vi "Insert_test.vi"(7 "Added time":refnum<vi>, 8 "error in (no error)":errorcluster, 9 "Sorted hits":T2, 10 "Bottom hit charts":T1, 11 "Top hit charts":T1) -> (0 "error out":errorcluster)   [LabVIEW 2016]
uses:
  Typedefs/Hit chart cluster refnum.ctl
  Global Variables/Global Resolution.vi
panel:
  out "Numeric":u64
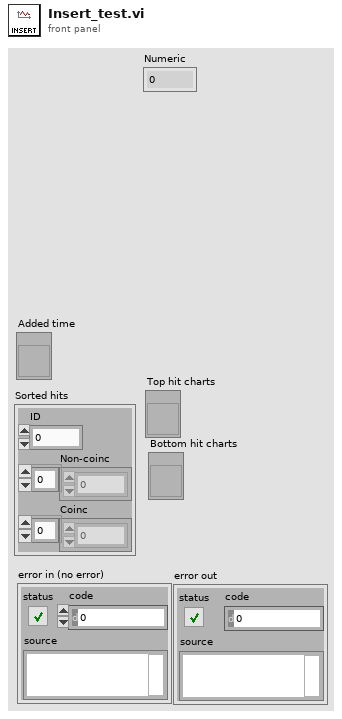
[diagram p1: front panel]
types:
  T1 = typedef "Hit chart cluster refnum.ctl" = refnum<vi>
  T2 = cluster{"ID":i8, "Non-coinc":u64[], "Coinc":u64[]}
  T3 = typedef "HitChart refnum.ctl" = refnum<vi>
  T4 = typedef "HitChart.ctl" = cluster{"Waveform Chart":cluster{"Coincidences":dbl, "Non-coincidences":dbl, "Ratio":dbl, "Total hits":dbl}[], "Last update timestamp":timestamp, "Resolution(s)":dbl, "nondisplayed coincs":i32, "nondisplayed noncoincs":i32, "Last upd":i64, "ID":i8}
  T5 = cluster{"Coincidences":dbl, "Non-coincidences":dbl, "Ratio":dbl, "Total hits":dbl}
  T6 = cluster{"Coincidences":dbl, "Non-coincidences":dbl, "Ratio":dbl, "Total hits":dbl}[]
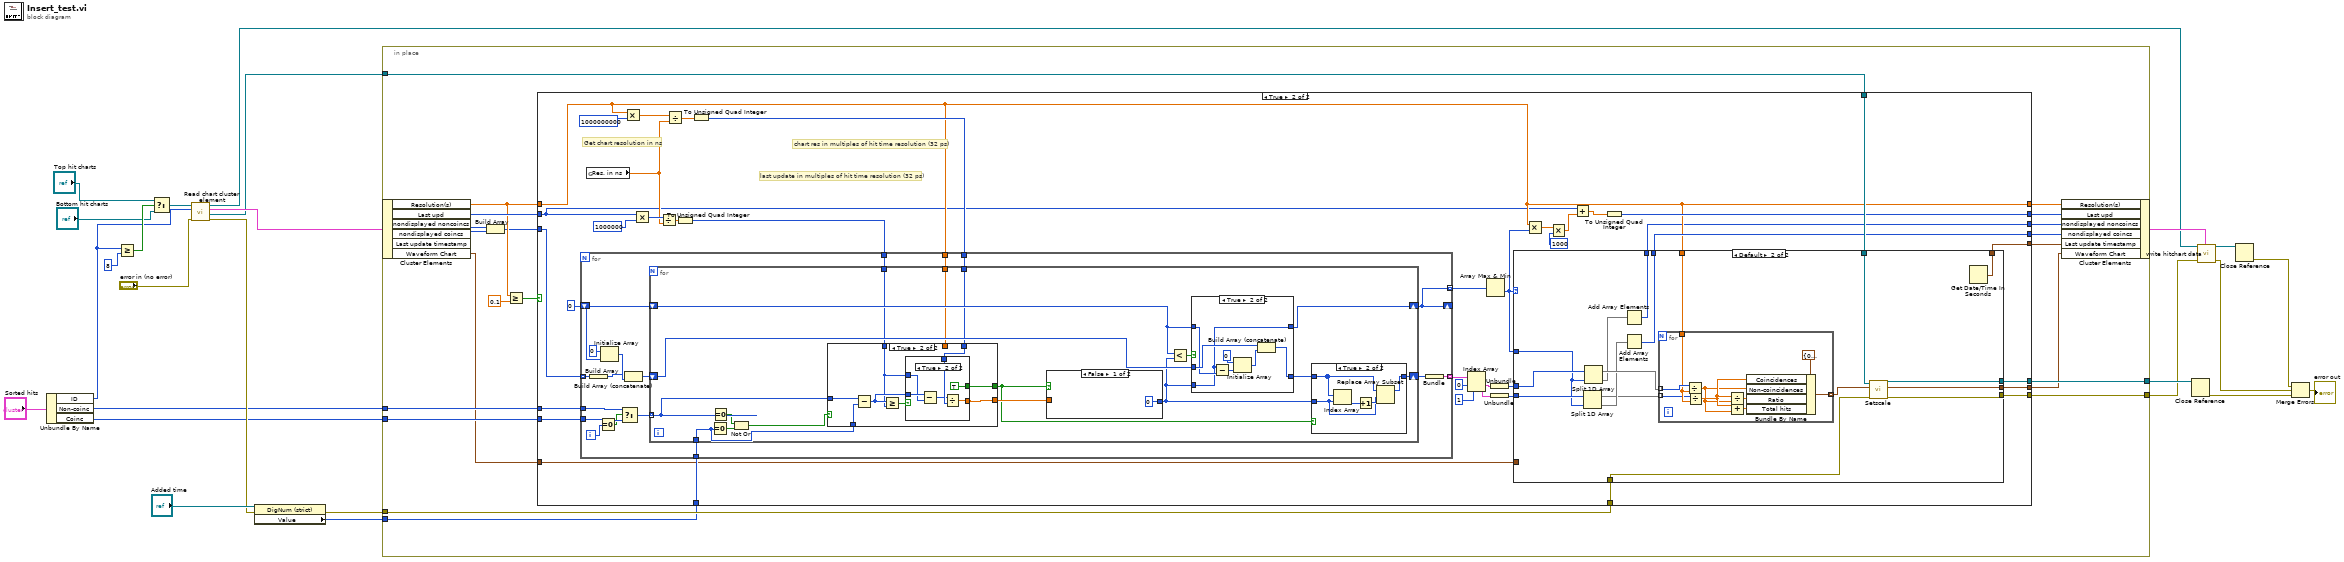
[diagram p0: block diagram]
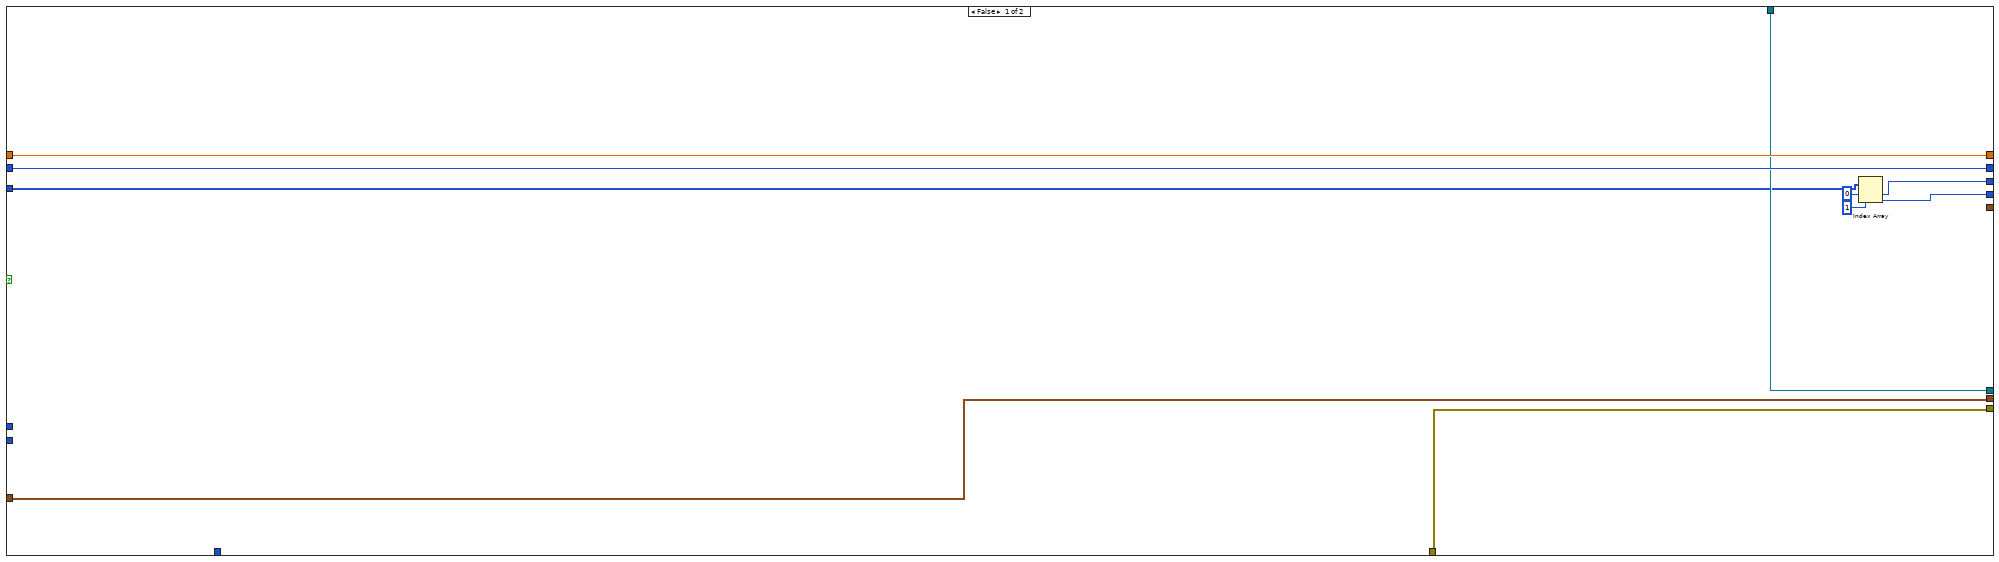
[diagram p2: hidden frame]
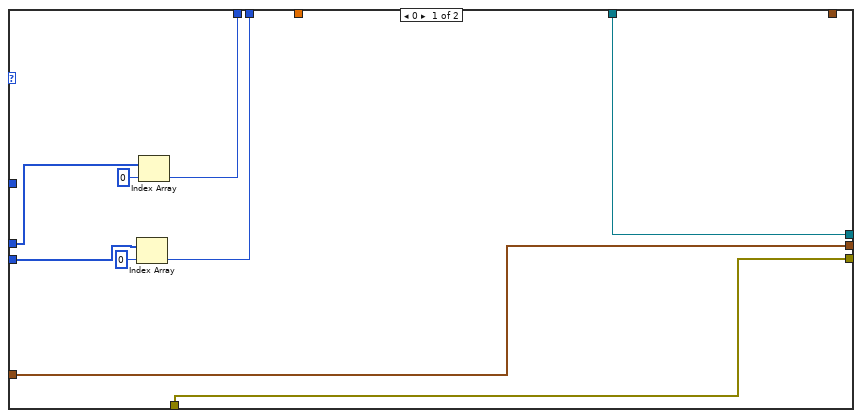
[diagram p3: hidden frame]
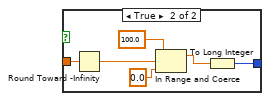
[diagram p4: hidden frame]
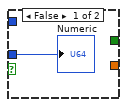
[diagram p6: hidden frame]
diagram:
  n1 = Unbundle By Name("Sorted hits") -> ("ID"=w21:i8, "Non-coinc"=w2:u64[], "Coinc"=w1:u64[])
  n2 = Greater Or Equal?(x=w21, y=i8 8) -> (x >= y?=w22:bool)
  n3 = Select(t="Top hit charts", s=w22, f="Bottom hit charts") -> (s? t:f=w23:T1)
  n4 = call "Read chart cluster element.vi"("error in (no error)"="error in (no error)", "Channel"=w21, "Chart cluster"=w23) -> ("error out"=w7:errorcluster, "Chart ref"=w19:T3, 2:"Chart cluster"=w20:T4, 3:"Chart cluster"=w11:T1)  [unwired: 5 in]
  n5 = property class="DigNum (strict)"(reference="Added time", error in=w7) -> (error out=w6:errorcluster, "Value"=w5:u64)  [unwired: 1 out]
  n6 = in-place {
    in-place-border: w2 -> [w46]
    in-place-border: w1 -> [w45]
    in-place-border: w19 -> [w44]
    in-place-border: [w42] -> w17
    in-place-border: w6 -> [w41]
    in-place-border: [w38] -> w14
    in-place-border: w5 -> [w33]
    n7 = in-place-cluster #1(w20) -> ("Resolution(s)"=w34:dbl, "Last upd"=w40:i64, "nondisplayed noncoincs"=w32:i32, "nondisplayed coincs"=w31:i32, "Waveform Chart"=w26:T6)  [unwired: 1 out]
    n8 = Build Array(w32, w31) -> (w30:i32[])
    n9 = Greater Or Equal?(x=w34, y=0.1) -> (x >= y?=w37:bool)
    n10 = case shown="True" w37 {
      tunnel: w46 -> [_ w95]
      tunnel: w30 -> [w52 w71]
      tunnel: w45 -> [_ w92]
      tunnel: w44 -> [w53 w91]
      tunnel: [w48 w90] -> w43
      tunnel: [w53 w89] -> w42
      tunnel: w41 -> [w56 w88]
      tunnel: w40 -> [w54 w72]
      tunnel: [w54 w76] -> w39
      tunnel: w34 -> [w55 w73]
      tunnel: [w56 w87] -> w38
      tunnel: [w55 w73] -> w35
      tunnel: w33 -> [_ w75]
      tunnel: [w49 w70] -> w29
      tunnel: [_ w59] -> w28
      tunnel: [w47 w58] -> w27
      tunnel: w26 -> [w47 w57]
      frame False {
        n11 = Index Array(array=w52, index #1=0 ("index"), index #2=1 ("index")) -> (element #1=w49:i32, element #2=w48:i32)
      }
      frame True {
        # "last update in multiples of hit time resolution (32 ps)"
        # "chart res in multiples of hit time resolution (32 ps)"
        # "Get chart resolution in ns"
        n12 = global read "Global Resolution.vi" "Res. in ns"() -> (w74:ext)
        n13 = Multiply(x=w73, y=i64 1000000000) -> (x*y=w83:dbl)
        n14 = Multiply(x=w72, y=i64 1000000) -> (x*y=w82:i64)
        n15 = Divide(x=w82, y=w74) -> (x/y=w81:ext)
        n16 = Divide(x=w83, y=w74) -> (x/y=w79:ext)
        n17 = To Unsigned Quad Integer(1:w81) -> (0:w80:u64)
        n18 = To Unsigned Quad Integer(1:w79) -> (0:w78:u64)
        n19 = for {
          tunnel: w80 -> [w148]
          tunnel: w78 -> [w147]
          tunnel: w95 -> [w145]
          tunnel: w92 -> [w144]
          shift-right: [w133] -> _
          shift-left: 0 -> [w141]
          tunnel: w75 -> [w139]
          tunnel: w73 -> [w135]
          tunnel: w71 -> [w134] mode=indexing
          tunnel: [w133] -> w69 mode=indexing
          tunnel: [w131] -> w68 mode=indexing
          i -> [w146]
          n20 = Build Array(w134) -> (w138:i32[])
          n21 = Equal To 0?(x=w146) -> (x = 0?=w137:bool)
          n22 = Initialize Array(0, w141) -> (w142:i32[])
          n23 = Select(t=w145, s=w137, f=w144) -> (s? t:f=w143:u64[])
          n24 = Build Array (concatenate)(w138, w142) -> (w136:i32[])
          n25 = for {
            tunnel: w143 -> [w154] mode=indexing
            tunnel: w148 -> [w157]
            tunnel: w147 -> [w158]
            shift-right: [w164] -> w132
            shift-left: w136 -> [w165]
            shift-right: [w163] -> w133
            shift-left: w141 -> [w162]
            tunnel: w139 -> [w149]
            tunnel: w135 -> [w155]
            n26 = Equal To 0?(x=w149) -> (x = 0?=w152:bool)
            n27 = Equal To 0?(x=w154) -> (x = 0?=w151:bool)
            n28 = Not Or(1:w152, 2:w151) -> (0:w150:bool)
            n29 = case shown="True" w150 {
              tunnel: [_ w178] -> w159
              tunnel: w158 -> [_ w180]
              tunnel: w157 -> [_ w175]
              tunnel: w154 -> [_ w179]
              tunnel: w155 -> [_ _]
              tunnel: [_ w174] -> w153
              tunnel: w149 -> [_ w173]
              frame False {
              }
              frame True {
                n30 = Subtract(x=w179, y=w173) -> (x-y=w176:u64)
                n31 = Greater Or Equal?(x=w176, y=w175) -> (x >= y?=w177:bool)
                n32 = case shown="True" w177 {
                  tunnel: w180 -> [_ w187]
                  tunnel: [_ w186] -> w178
                  tunnel: w176 -> [w181 w184]
                  tunnel: w175 -> [_ w183]
                  tunnel: [_ TRUE] -> w174
                  frame False {
                    "Numeric" <- w181
                  }
                  frame True {
                    n33 = Subtract(x=w184, y=w183) -> (x-y=w185:u64)
                    n34 = Divide(x=w185, y=w187) -> (x/y=w186:dbl)
                  }
                }
              }
            }
            n35 = case shown="False" w153 {
              tunnel: w159 -> [_ w172]
              tunnel: [0 w171] -> w156
              frame False {
              }
              frame True {
                n36 = Round Toward -Infinity(1:w172) -> (0:w169:dbl)
                n37 = In Range and Coerce(upper limit=100.0, x=w169, lower limit=0.0) -> (coerced(x)=w170:dbl)  [unwired: 1 out]
                n38 = To Long Integer(number=w170) -> (32bit integer=w171:i32)
              }
            }
            n39 = Less?(x=w162, y=w156) -> (x < y?=w160:bool)
            n40 = case shown="True" w160 {
              tunnel: w165 -> [w195 w200]
              tunnel: [w195 w201] -> w161
              tunnel: w162 -> [w194 w198]
              tunnel: w156 -> [_ w196]
              tunnel: [w194 w196] -> w163
              frame False {
              }
              frame True {
                n41 = Subtract(x=w196, y=w198) -> (x-y=w197:i32)
                n42 = Initialize Array(0, w197) -> (w199:i32[])
                n43 = Build Array (concatenate)(w200, w199) -> (w201:i32[])
              }
            }
            n44 = case shown="True" w153 {
              tunnel: [w188 w193] -> w164
              tunnel: w161 -> [w188 w190]
              tunnel: w156 -> [_ w189]
              frame False {
              }
              frame True {
                n45 = Index Array(array=w190, index=w189) -> (element=w192:i32)
                n46 = Increment(x=w192) -> (x+1=w191:i32)
                n47 = Replace Array Subset(array=w190, new element=w191, index=w189) -> (w193:i32[])
              }
            }
          }
          n48 = Bundle(w132) -> (w131:cluster{i32[]})  [unwired: 1 in]
        }
        n49 = Index Array(array=w68, index #1=0 ("index"), index #2=1 ("index")) -> (element #1=w64:cluster{i32[]}, element #2=w63:cluster{i32[]})
        n50 = Array Max & Min(array=w69) -> (min value=w61:i32)  [unwired: 3 out]
        n51 = Unbundle(w64) -> (w65:i32[])
        n52 = Unbundle(w63) -> (w62:i32[])
        n53 = case shown="Default" w61 {
          tunnel: w91 -> [w98 w121]
          tunnel: w65 -> [w104 w115]
          tunnel: w62 -> [w101 w114]
          tunnel: [w100 w120] -> w70
          tunnel: [w99 w119] -> w90
          tunnel: [w98 w118] -> w89
          tunnel: w88 -> [w97 w117]
          tunnel: [w97 w116] -> w87
          tunnel: w73 -> [_ w113]
          tunnel: w61 -> [_ w112]
          tunnel: [_ w106] -> w59
          tunnel: [w96 w105] -> w58
          tunnel: w57 -> [w96 _]
          frame 0 {
            n54 = Index Array(array=w101, index=0) -> (element=w99:i32)
            n55 = Index Array(array=w104, index=0) -> (element=w100:i32)
          }
          frame Default {
            n56 = Split 1D Array(array=w114, index=w112) -> (first subarray=w107:i32[], second subarray=w108:i32[])
            n57 = Split 1D Array(array=w115, index=w112) -> (first subarray=w111:i32[], second subarray=w109:i32[])
            n58 = Add Array Elements(numeric array=w109) -> (sum=w120:i32)
            n59 = Add Array Elements(numeric array=w108) -> (sum=w119:i32)
            n60 = for {
              tunnel: w111 -> [w127] mode=indexing
              tunnel: w113 -> [w126]
              tunnel: [w123] -> w110 mode=indexing
              tunnel: w107 -> [w122] mode=indexing
              n61 = Divide(x=w127, y=w126) -> (x/y=w124:dbl)
              n62 = Divide(x=w122, y=w126) -> (x/y=w125:dbl)
              n63 = Divide(x=w125, y=w124) -> (x/y=w130:dbl)
              n64 = Add(x=w125, y=w124) -> (x+y=w129:dbl)
              n65 = Bundle By Name(cluster=T5 {"Coincidences"=0.0, "Non-coincidences"=0.0, "Ratio"=0.0, "Total hits"=0.0} ("Waveform Chart"), "Coincidences"=w125, "Non-coincidences"=w124, "Ratio"=w130, "Total hits"=w129) -> (w123:T5)
            }
            n66 = call "Setscale.vi"("error in (no error)"=w117, "Array"=w110, "WaveformChart in"=w121) -> ("error out"=w116:errorcluster, "Value"=w105:T6, "WaveformChart out"=w118:T3)  [unwired: 6 in]
            n67 = Get Date/Time In Seconds() -> (seconds since 1Jan1904=w106:timestamp)
          }
        }
        n68 = Multiply(x=w73, y=w61) -> (x*y=w60:dbl)
        n69 = Multiply(x=w60, y=1000) -> (x*y=w84:dbl)
        n70 = Add(x=w72, y=w84) -> (x+y=w77:dbl)
        n71 = To Unsigned Quad Integer(1:w77) -> (0:w76:u64)
      }
    }
    n72 = in-place-cluster #1("Resolution(s)"=w35, "Last upd"=w39, "nondisplayed noncoincs"=w29, "nondisplayed coincs"=w43, "Last update timestamp"=w28, "Waveform Chart"=w27) -> (w15:T4)
  }
  n73 = Close Reference(reference=w17) -> (error out=w12:errorcluster)  [unwired: 1 in]
  n74 = call "write hitchart data.vi"("Histogram cluster"=w15, "error in (no error)"=w14, "Hit charts"=w11) -> ("error out"=w13:errorcluster, "Hit charts"=w10:T1)  [unwired: 7 in]
  n75 = Close Reference(reference=w10) -> (error out=w9:errorcluster)  [unwired: 1 in]
  n76 = Merge Errors(w9, w13, w12) -> (→"error out":errorcluster)
